vi "ReadTriggerInputNode.vi"(8 "Error In":errorcluster, 11 "Keithley2602 Node In":refnum<k20>) -> (0 "Error Out":errorcluster, 2 "Trigger Input Configuration":T1={"Type"=enum."None", "Timeout (ms)"=100, "Delay (ms)"=0, "Digital IO Line (1-14)"=1, "Digital IO Mode"=enum."Falling"}, 3 "Keithley2602 Node Out":refnum<k20>)   [LabVIEW 2013]
uses:
  TriggerInputConfiguration.ctl
  TriggerInputType.ctl
  driver/Public/Controls/TriggerMode.ctl
  driver/Keithley-2602.lvlib
  <vilib>/xml/NI_XML.lvlib
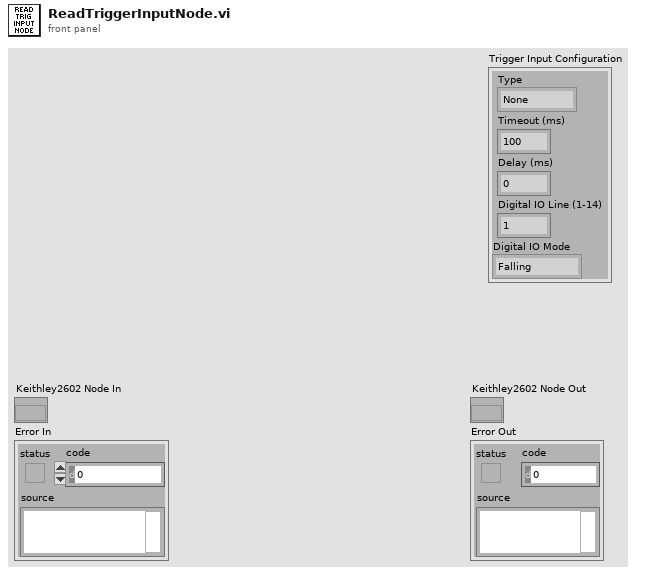
[diagram p1: front panel]
types:
  T1 = typedef "TriggerInputConfiguration.ctl" = cluster{"Type":T2, "Timeout (ms)":u32, "Delay (ms)":u32, "Digital IO Line (1-14)":u8, "Digital IO Mode":T3}
  T2 = typedef "TriggerInputType.ctl" = enum16{"None", "Digital IO", "Bus"}
  T3 = typedef "Keithley-2602.lvlib/TriggerMode.ctl" = enum16{"Falling", "Rising", "Either", "Synchronous"}
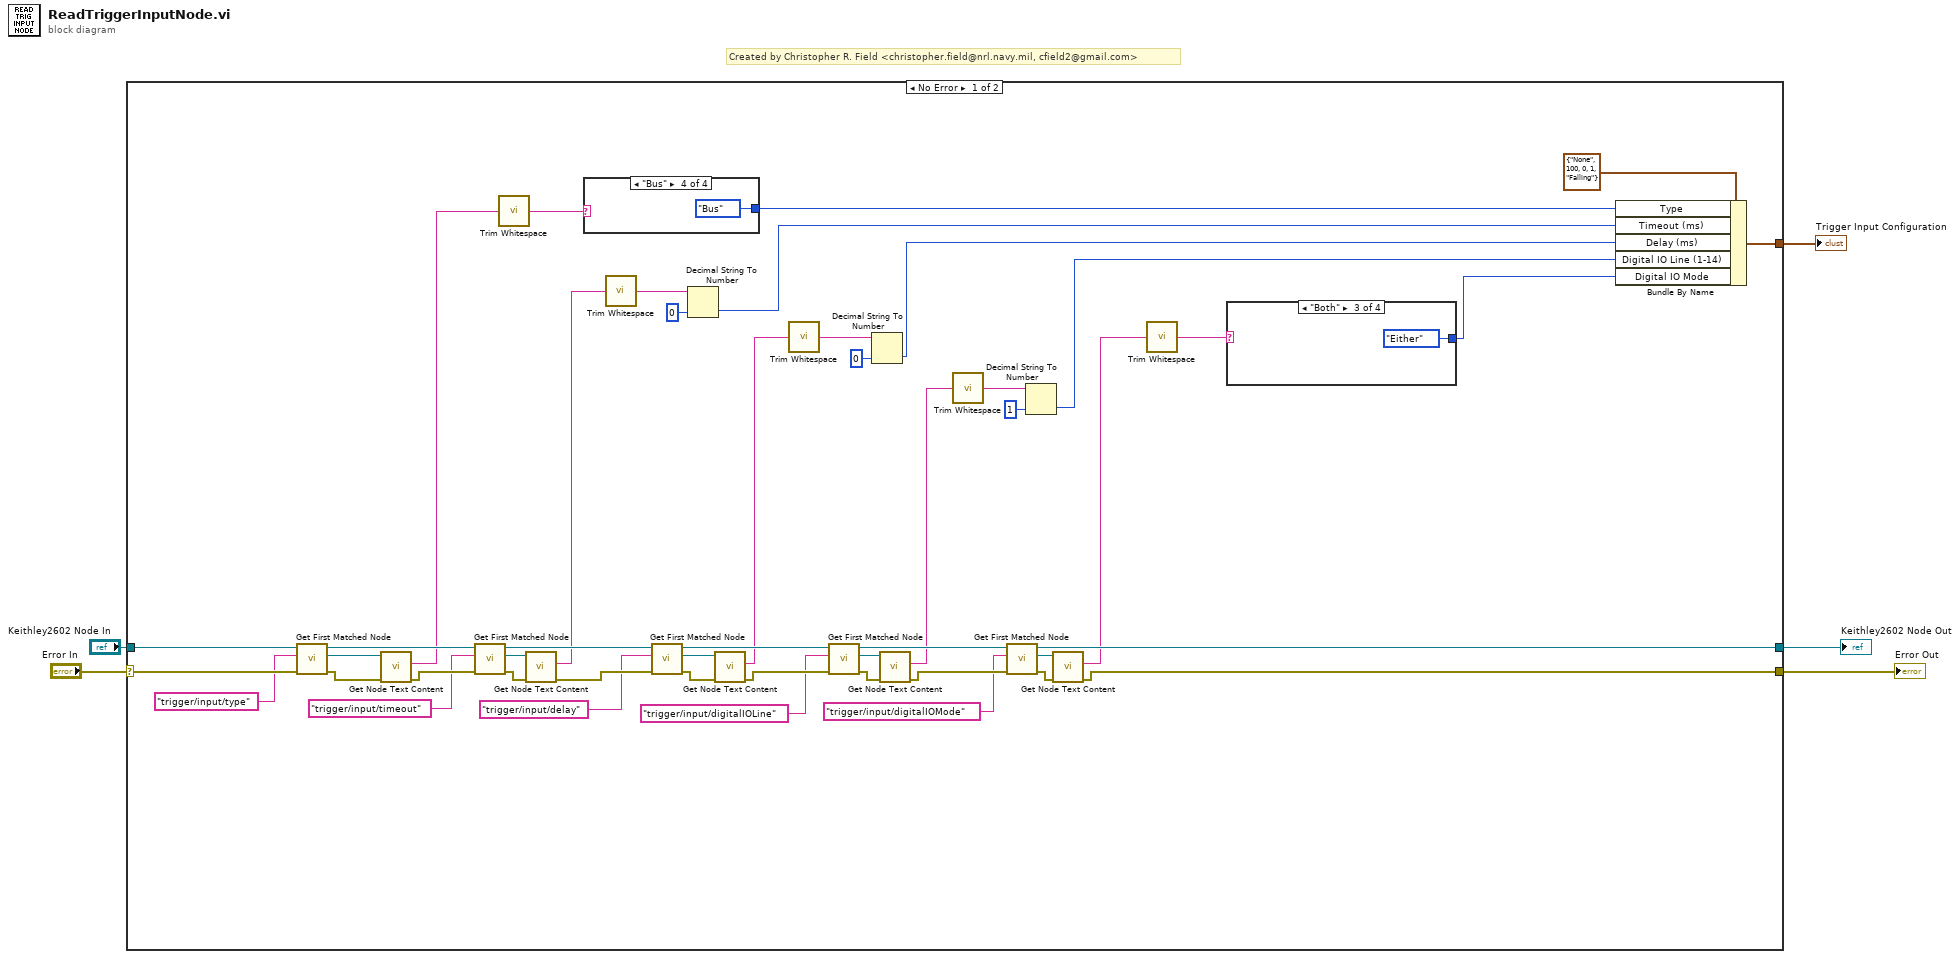
[diagram p0: block diagram]
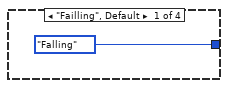
[diagram p2: hidden frame]
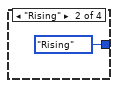
[diagram p3: hidden frame]
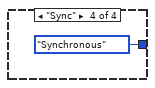
[diagram p4: hidden frame]
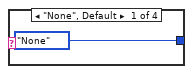
[diagram p5: hidden frame]
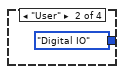
[diagram p6: hidden frame]
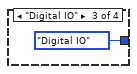
[diagram p7: hidden frame]
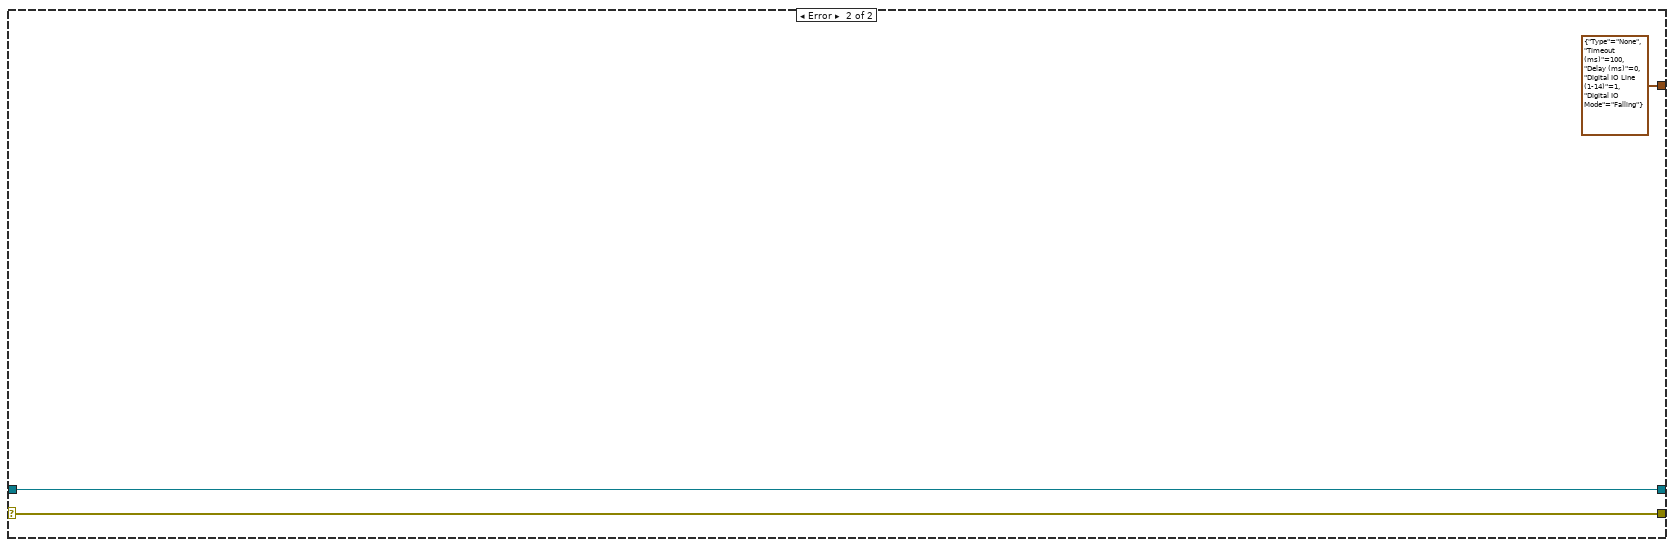
[diagram p8: hidden frame]
diagram:
  # "Created by Christopher R. Field <christopher.field@nrl.navy.mil, cfield2@gmail.com>"
  n1 = case shown="No Error" "Error In" {
    selector: "Error In" -> [w50 w62]
    tunnel: "Keithley2602 Node In" -> [w51 w63]
    tunnel: [w19 w63] -> w3
    tunnel: [w18 w62] -> w2
    tunnel: [w52 T1 {"Type"=enum."None", "Timeout (ms)"=100, "Delay (ms)"=0, "Digital IO Line (1-14)"=1, "Digital IO Mode"=enum."Falling"} ("Trigger Input Configuration")] -> w1
    frame No Error {
      n2 = call <vilib>:"Get First Matched Node.vi"("error in (no error)"=w50, "XPath expression"="trigger/input/type", "node in"=w51) -> ("error out"=w47:errorcluster, "node result"=w48:refnum<k20>, "node out"=w45:refnum<k20>)  [unwired: 6 in]
      n3 = call <vilib>:"Get Node Text Content.vi"("error in (no error)"=w47, "node in"=w48) -> ("error out"=w44:errorcluster, "node text"=w15:string)  [unwired: 7 in, 1 out]
      n4 = call <vilib>:"Get First Matched Node.vi"("error in (no error)"=w44, "XPath expression"="trigger/input/timeout", "node in"=w45) -> ("error out"=w42:errorcluster, "node result"=w43:refnum<k20>, "node out"=w38:refnum<k20>)  [unwired: 6 in]
      n5 = call <vilib>:"Trim Whitespace.vi"("string"=w15) -> ("trimmed string"=w16:string)  [unwired: 1 in]
      n6 = call <vilib>:"Get Node Text Content.vi"("error in (no error)"=w42, "node in"=w43) -> ("error out"=w37:errorcluster, "node text"=w13:string)  [unwired: 7 in, 1 out]
      n7 = case shown="\"Bus\"" w16 {
        tunnel: [TriggerInputType."None" ("Type") TriggerInputType."Digital IO" ("Type") TriggerInputType."Digital IO" ("Type") TriggerInputType."Bus" ("Type")] -> w46
        frame "None", Default {
        }
        frame "User" {
        }
        frame "Digital IO" {
        }
        frame "Bus" {
        }
      }
      n8 = call <vilib>:"Trim Whitespace.vi"("string"=w13) -> ("trimmed string"=w14:string)  [unwired: 1 in]
      n9 = call <vilib>:"Get First Matched Node.vi"("error in (no error)"=w37, "XPath expression"="trigger/input/delay", "node in"=w38) -> ("error out"=w35:errorcluster, "node result"=w36:refnum<k20>, "node out"=w31:refnum<k20>)  [unwired: 6 in]
      n10 = Decimal String To Number(string=w14, default (0L)=u32 0 ("default (0 I32)")) -> (number=w39:u32)  [unwired: 1 in, 1 out]
      n11 = call <vilib>:"Get Node Text Content.vi"("error in (no error)"=w35, "node in"=w36) -> ("error out"=w30:errorcluster, "node text"=w11:string)  [unwired: 7 in, 1 out]
      n12 = call <vilib>:"Trim Whitespace.vi"("string"=w11) -> ("trimmed string"=w12:string)  [unwired: 1 in]
      n13 = call <vilib>:"Get First Matched Node.vi"("error in (no error)"=w30, "XPath expression"="trigger/input/digitalIOLine", "node in"=w31) -> ("error out"=w27:errorcluster, "node result"=w28:refnum<k20>, "node out"=w24:refnum<k20>)  [unwired: 6 in]
      n14 = Decimal String To Number(string=w12, default (0L)=u32 0 ("default (0 I32)")) -> (number=w32:u32)  [unwired: 1 in, 1 out]
      n15 = call <vilib>:"Get Node Text Content.vi"("error in (no error)"=w27, "node in"=w28) -> ("error out"=w23:errorcluster, "node text"=w9:string)  [unwired: 7 in, 1 out]
      n16 = call <vilib>:"Trim Whitespace.vi"("string"=w9) -> ("trimmed string"=w10:string)  [unwired: 1 in]
      n17 = call <vilib>:"Get First Matched Node.vi"("error in (no error)"=w23, "XPath expression"="trigger/input/digitalIOMode", "node in"=w24) -> ("error out"=w20:errorcluster, "node result"=w21:refnum<k20>, "node out"=w19:refnum<k20>)  [unwired: 6 in]
      n18 = Decimal String To Number(string=w10, default (0L)=u32 1 ("default (0 I32)")) -> (number=w25:u32)  [unwired: 1 in, 1 out]
      n19 = call <vilib>:"Get Node Text Content.vi"("error in (no error)"=w20, "node in"=w21) -> ("error out"=w18:errorcluster, "node text"=w7:string)  [unwired: 7 in, 1 out]
      n20 = call <vilib>:"Trim Whitespace.vi"("string"=w7) -> ("trimmed string"=w8:string)  [unwired: 1 in]
      n21 = case shown="\"Both\"" w8 {
        tunnel: [TriggerMode."Falling" ("Digital IO Mode") TriggerMode."Rising" ("Digital IO Mode") TriggerMode."Either" ("Digital IO Mode") TriggerMode."Synchronous" ("Digital IO Mode")] -> w17
        frame "Failling", Default {
        }
        frame "Rising" {
        }
        frame "Both" {
        }
        frame "Sync" {
        }
      }
      n22 = Bundle By Name(cluster=T1 {"Type"=enum."None", "Timeout (ms)"=100, "Delay (ms)"=0, "Digital IO Line (1-14)"=1, "Digital IO Mode"=enum."Falling"} ("Trigger Input Configuration"), "Type"=w46, "Timeout (ms)"=w39, "Delay (ms)"=w32, "Digital IO Line (1-14)"=w25, "Digital IO Mode"=w17) -> (w52:T1)
    }
    frame Error {
    }
  }
  "Keithley2602 Node Out" <- w3
  "Error Out" <- w2
  "Trigger Input Configuration" <- w1
